vi "CryoServer Close.vi"(8 "error in (no error)":errorcluster, 11 "CryoServer in":refnum<class "CryoServer.lvclass">) -> (0 "error out":errorcluster, 3 "CryoServer out":refnum<class "CryoServer.lvclass">)   [LabVIEW 2021, in "CryoServer.lvclass"]
uses:
  CryoServer.lvclass
  CryoServer.lvclass/CryoServer.ctl
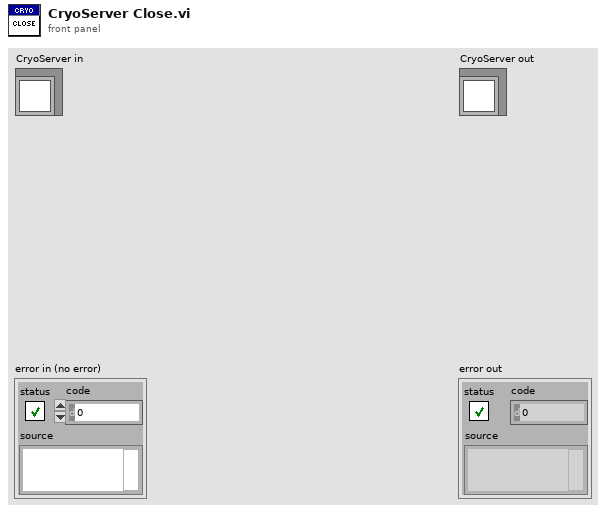
[diagram p1: front panel]
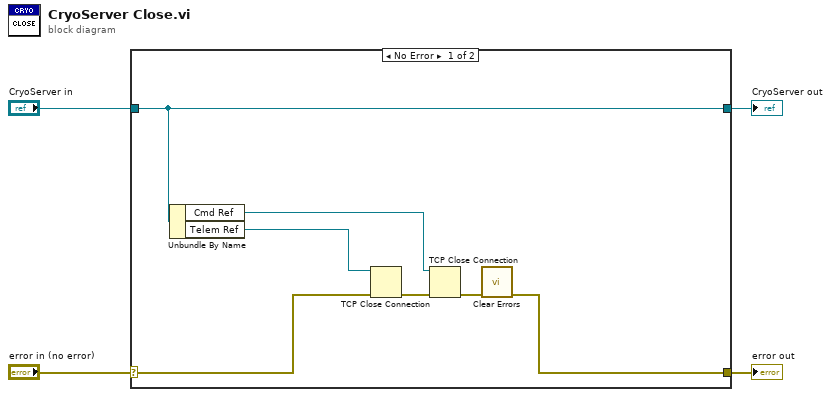
[diagram p0: block diagram]
diagram:
  n1 = case shown="No Error" "error in (no error)" {
    selector: "error in (no error)" -> [w8 w13]
    tunnel: [w5 w13] -> w3
    tunnel: [w11 w12] -> w1
    tunnel: "CryoServer in" -> [w11 w12]
    frame No Error {
      n2 = Unbundle By Name(w11) -> ("Cmd Ref"=w9:refnum<k5>, "Telem Ref"=w10:refnum<k5>)
      n3 = TCP Close Connection(connection ID=w10, error in (no error)=w8) -> (error out=w7:errorcluster)  [unwired: 1 in, 1 out]
      n4 = TCP Close Connection(connection ID=w9, error in (no error)=w7) -> (error out=w6:errorcluster)  [unwired: 1 in, 1 out]
      n5 = call <vilib>:"Clear Errors.vi"("error in (no error)"=w6) -> ("error out"=w5:errorcluster)  [unwired: 5 in, 1 out]
    }
    frame Error {
    }
  }
  "error out" <- w3
  "CryoServer out" <- w1
